vi "MH_BufferRecordV2.vi"(6 "WindowWidth":i32, 7 "truetime":u64, 8 "WinIndex":i32, 9 "Buffindex":i32, 10 "Buffsize":i32, 11 "Buffer":u64[](array[numeric])) -> (0 "WinIndexOut":i32, 1 "BuffIndexOut":i32, 2 "NewBuffsize":i32, 3 "tableau (n rotations)":u64[](array[numeric]))   [LabVIEW 2019]
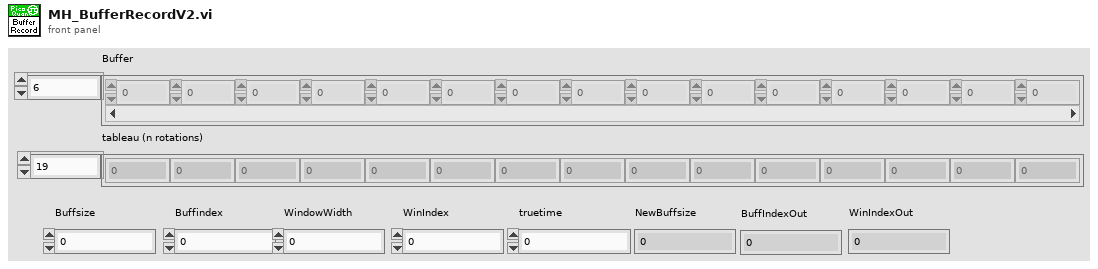
[diagram p1: front panel]
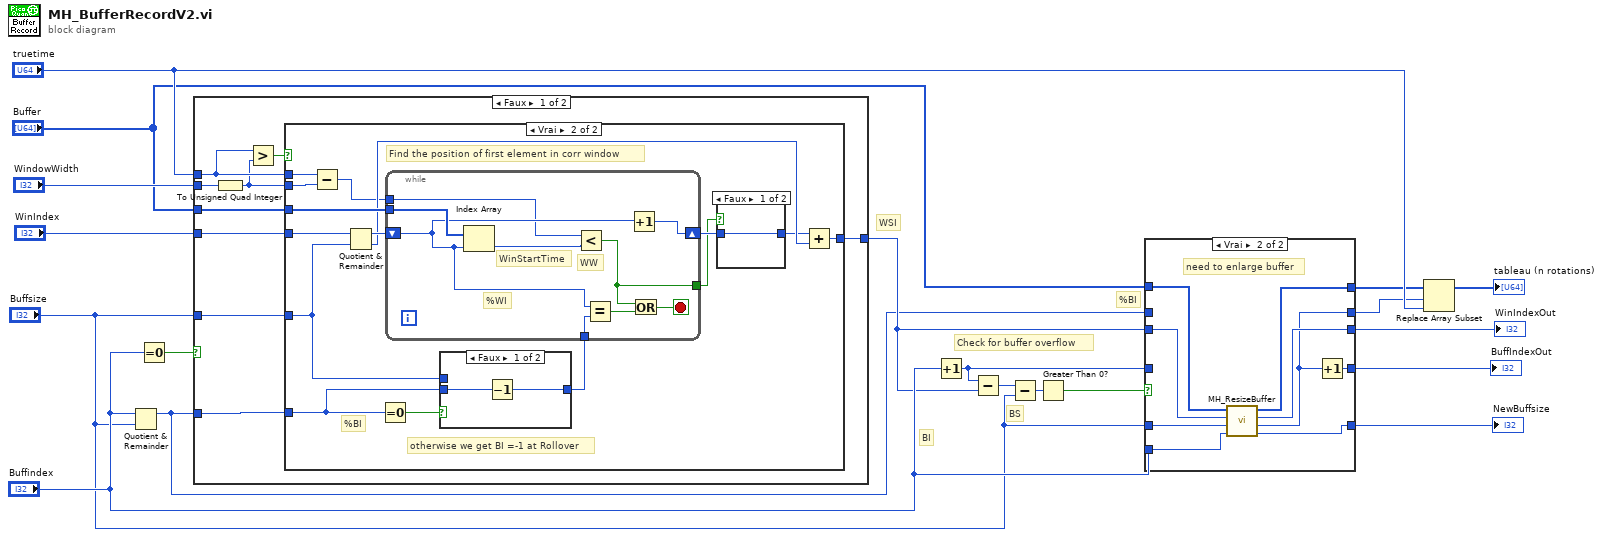
[diagram p0: block diagram]
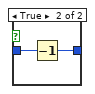
[diagram p3: hidden frame]
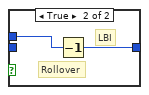
[diagram p4: hidden frame]
diagram:
  # "%BI"
  # "BS"
  # "Check for buffer overflow"
  # "WSI"
  # "BI"
  n1 = Quotient & Remainder(x="Buffindex", y="Buffsize") -> (x-y*floor(x/y)=w2:i32)  [unwired: 1 out]
  n2 = Equal To 0?(x="Buffindex") -> (x = 0?=w5:bool)
  n3 = case shown="Faux" w5 {
    tunnel: "truetime" -> [w23 _]
    tunnel: "WinIndex" -> [w24 w61]
    tunnel: "WindowWidth" -> [w22 _]
    tunnel: "Buffer" -> [w28 _]
    tunnel: [w25 w61] -> w7
    tunnel: "Buffsize" -> [w26 _]
    tunnel: w2 -> [w27 _]
    frame False {
      n4 = To Unsigned Quad Integer(1:w22) -> (0:w21:u64)
      n5 = Greater?(x=w23, y=w21) -> (0:w20:bool)
      n6 = case shown="Vrai" w20 {
        tunnel: w28 -> [_ w44]
        tunnel: w27 -> [_ w33]
        tunnel: w26 -> [_ w32]
        tunnel: [w29 w39] -> w25
        tunnel: w24 -> [w29 w38]
        tunnel: w23 -> [_ w36]
        tunnel: w21 -> [_ w35]
        frame False {
          # "All records will be in window"
        }
        frame True {
          # "Find the position of first element in corr window"
          # "otherwise we get BI =-1 at Rollover"
          # "%BI"
          n7 = Subtract(x=w36, y=w35) -> (x-y=w34:u64)
          n8 = Quotient & Remainder(x=w38, y=w32) -> (x-y*floor(x/y)=w40:i32, floor(x/y)=w37:i32)
          n9 = Equal To 0?(x=w33) -> (x = 0?=w41:bool)
          n10 = case shown="Faux" w41 {
            tunnel: w33 -> [w58 _]
            tunnel: [w57 w59] -> w42
            tunnel: w32 -> [_ w60]
            frame False {
              n11 = Decrement(x=w58) -> (x-1=w57:i32)
            }
            frame True {
              # "LBI"
              # "Rollover"
              n12 = Decrement(x=w60) -> (x-1=w59:i32)
            }
          }
          n13 = while {
            tunnel: w34 -> [w49]
            tunnel: w44 -> [w56]
            shift-right: [w53] -> w43
            shift-left: w40 -> [w51]
            tunnel: w42 -> [w54]
            tunnel: [w48] -> w30
            stop <- w55 stop-if-true
            # "WW"
            # "%WI"
            # "WinStartTime"
            n14 = Index Array(array=w56, index=w51) -> (element=w50:u64)
            n15 = Less?(x=w49, y=w50) -> (x < y?=w48:bool)
            n16 = Equal?(x=w51, y=w54) -> (x = y?=w52:bool)
            n17 = Increment(x=w51) -> (x+1=w53:i32)
            n18 = Or(x=w48, y=w52) -> (x .or. y?=w55:bool)
          }
          n19 = case shown="Faux" w30 {
            tunnel: w43 -> [w45 w47]
            tunnel: [w45 w46] -> w31
            frame False {
            }
            frame True {
              n20 = Decrement(x=w47) -> (x-1=w46:i32)
            }
          }
          n21 = Add(x=w31, y=w37) -> (x+y=w39:i32)
        }
      }
    }
    frame True {
      # "no need to check WSI"
      # "BufferIndex = 0"
    }
  }
  n22 = Increment(x="Buffindex") -> (x+1=w4:i32)
  n23 = Subtract(x=w4, y=w7) -> (x-y=w11:i32)
  n24 = Subtract(x=w11, y="Buffsize") -> (x-y=w10:i32)
  n25 = Greater Than 0?(x=w10) -> (x > 0?=w8:bool)
  n26 = case shown="Vrai" w8 {
    tunnel: "Buffer" -> [w64 w75]
    tunnel: "Buffsize" -> [w65 w72]
    tunnel: [w64 w74] -> w9
    tunnel: "Buffindex" -> [_ w73]
    tunnel: w7 -> [w66 w71]
    tunnel: [w63 w68] -> w6
    tunnel: [w66 w70] -> w12
    tunnel: w2 -> [w63 _]
    tunnel: w4 -> [w62 _]
    tunnel: [w65 w69] -> w3
    tunnel: [w62 w67] -> w1
    frame False {
    }
    frame True {
      # "need to enlarge buffer"
      n27 = call <userlib>:"MH_ResizeBuffer.vi"("Buffindex"=w73, "Buffsize"=w72, "WinIndex"=w71, "Tableau"=w75) -> ("NewBuffsize"=w69:i32, "NewBuffIndex"=w68:i32, "NewWinIndex"=w70:i32, "tableau (n rotations)"=w74:u64[])  [unwired: 2 in, 2 out]
      n28 = Increment(x=w68) -> (x+1=w67:i32)
    }
  }
  "BuffIndexOut" <- w1
  "WinIndexOut" <- w12
  "NewBuffsize" <- w3
  n29 = Replace Array Subset(array=w9, new element="truetime", index=w6) -> (→"tableau (n rotations)":u64[])
